vi "Initialize Resources.vi"(7 "Custom Device Name":string, 8 "error in":errorcluster, 10 "Custom Device API in":refnum<class "Custom Device API.lvclass">, 11 "Custom Device in":refnum<class "SystemMonitor Engine.lvclass">) -> (0 "error out":errorcluster, 3 "Custom Device out":refnum<class "SystemMonitor Engine.lvclass">)   [LabVIEW 2026, in "SystemMonitor Engine.lvlib" / "SystemMonitor Engine.lvclass"]
uses:
  SystemMonitor Engine.lvclass
  <userlib>/Custom Device Interfaces_v1.lvlibp/CustomDeviceAPI/Custom Device API.lvclass
  SystemMonitor Engine.lvclass/SystemMonitor Engine.ctl
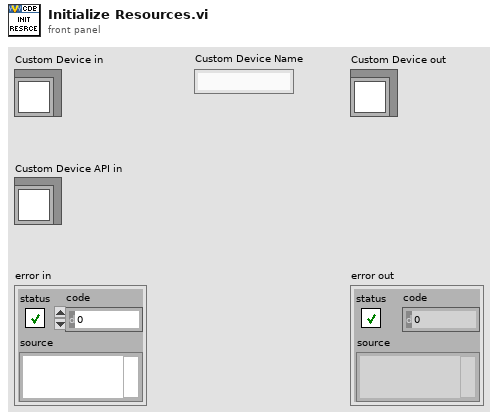
[diagram p1: front panel]
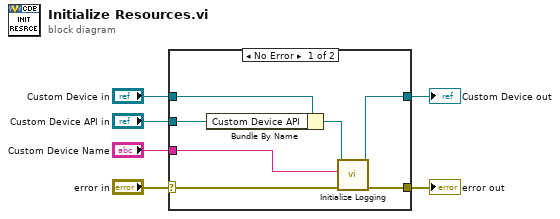
[diagram p0: block diagram]
diagram:
  n1 = case shown="No Error" "error in" {
    selector: "error in" -> [w13 w15]
    tunnel: [w12 w15] -> w5
    tunnel: [w11 w14] -> w3
    tunnel: "Custom Device in" -> [w9 w14]
    tunnel: "Custom Device Name" -> [w10 _]
    tunnel: "Custom Device API in" -> [w8 _]
    frame No Error {
      n2 = Bundle By Name(cluster=w9, "Custom Device API"=w8) -> (w7:refnum<class "SystemMonitor Engine.lvclass">)
      n3 = call "Initialize Logging.vi"("error in"=w13, "Custom Device Name"=w10, "Custom Device in"=w7) -> ("error out"=w12:errorcluster, "Custom Device out"=w11:refnum<class "SystemMonitor Engine.lvclass">)  [unwired: 7 in]
    }
    frame Error {
    }
  }
  "error out" <- w5
  "Custom Device out" <- w3
